vi "rs3 Get All Advanced3.vi"(7 "error in (no error)":errorcluster, 8 "device in":u64=370866768) -> (10 "ST_CensusEnable":cluster{"uDiameter":u32, "vDiameter":u32}={"uDiameter"=9, "vDiameter"=9}, 12 "ST_AE_Control":cluster{"meanIntensitySetpoint":u32}={"meanIntensitySetpoint"=400}, 14 "error":i32, 16 "Depth Table":T1={"depthUnits, um"=1000, "depthClampMin"=0, "depthClampMax"=65535, "disparityMultiplier"=0, "disparityShift"=0}, 17 "ST RAU vector":T7={"minWest"=1, "minEast"=1, "minWEsum"=1, "minNorth"=1, "minSouth"=1, "minNSSum"=1, "uStrink"=1, "vShrink"=1}, 18 "Dev out":u64=370866768, 19 "ST Color Control":T6, 20 "depth control":T2={"plusIncrement"=10, "MinusDecrement"=10, "deepSeaMedianThreshold"=528, "scoreThreshA"=10, "scoreThreshB"=1023, "textureDifferenceThreshold"=0, "textureCountThreshold"=0, "deepSeaSecondPeakThreshold"=27, "deepSeaNeighborThreshold"=20, "IrAgreeThreshold"=70}, 21 "STColorCorrection output":T9={"colorCorrection 1"=0.54785156, "colorCorrection 2"=0.32910156, "colorCorrection 3"=0.8222656, "colorCorrection 4"=0.109375, "colorCorrection 5"=-0.40527344, "colorCorrection 6"=-1.5253906, "colorCorrection 7"=0.95703125, "colorCorrection 8"=0.89160156, "colorCorrection 9"=0.7675781, "colorCorrection 10"=-0.4794922, "colorCorrection 11"=0.047851562, "colorCorrection 12"=-0.2705078}, 22 "HDAD":T10={"lambdaCensus"=26.0, "lambdaAD"=2100.0, "ignoreSAD"=0}, 23 "ST RSM":T8={"rsmBypass"=0, "diffThresh"=7.0, "sloRauDiffThresh"=3.0, "removeThresh"=33}, 24 "ST SLO Penalty":T3={"sloK1Penalty"=44, "sloK2Penalty"=502, "sloK1PenaltyMod1"=23, "sloK2PenaltyMod1"=237, "sloK1PenaltyMod2"=219, "sloK2PenaltyMod2"=113}, 25 "ST SLO Threshold":T4={"SLOdiffThresholdRed"=300, "SLODiffThresholdGreen"=300, "SLODiffThresholdBlue"=300}, 26 "ST Rau Threshold":T5={"rauDiffThresholdRed"=600, "rauDiffThresholdGreen"=600, "rauDiffThresholdBlue"=600}, 27 "error out":errorcluster)   [LabVIEW 2017, in "libRealSense3.lvlib"]
uses:
  libRealSense3.lvlib
panel:
  # "RS3 Get All Advanced"
  # "(C) 2017 Intel Corp.,  AGJ"
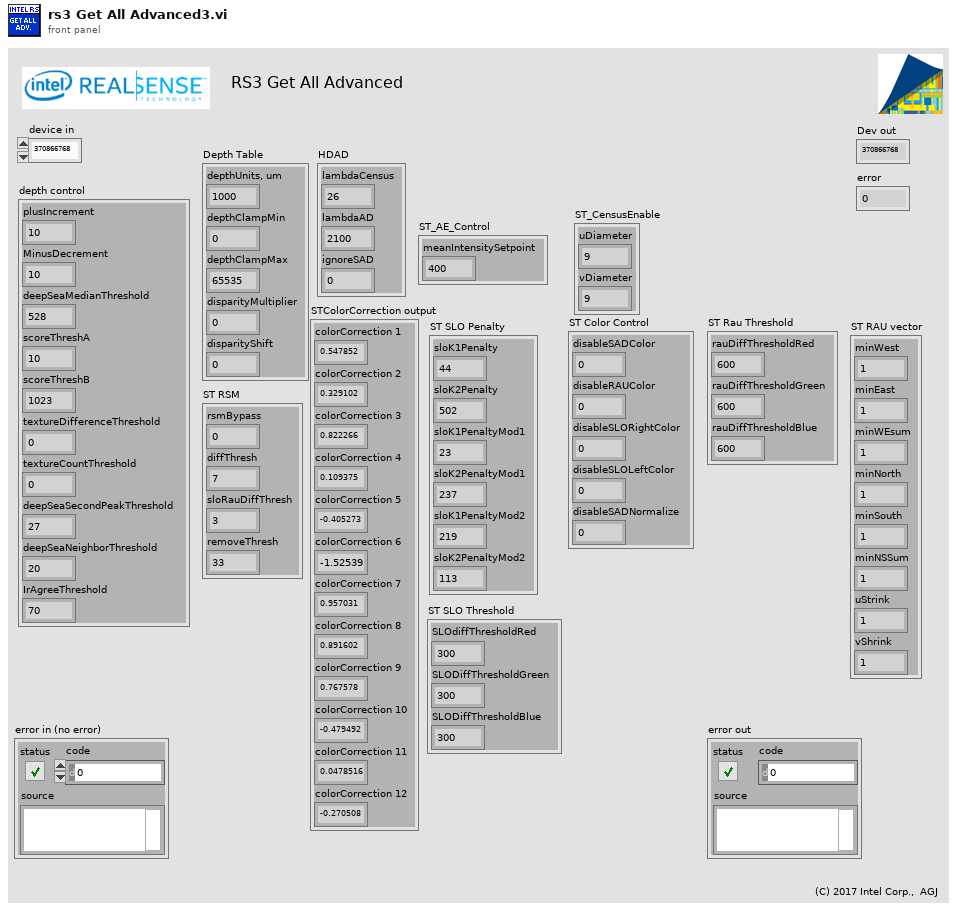
[diagram p1: front panel]
types:
  T1 = cluster{"depthUnits, um":u32, "depthClampMin":u32, "depthClampMax":u32, "disparityMultiplier":u32, "disparityShift":u32}
  T2 = cluster{"plusIncrement":u32, "MinusDecrement":u32, "deepSeaMedianThreshold":u32, "scoreThreshA":u32, "scoreThreshB":u32, "textureDifferenceThreshold":u32, "textureCountThreshold":u32, "deepSeaSecondPeakThreshold":u32, "deepSeaNeighborThreshold":u32, "IrAgreeThreshold":u32}
  T3 = cluster{"sloK1Penalty":u32, "sloK2Penalty":u32, "sloK1PenaltyMod1":u32, "sloK2PenaltyMod1":u32, "sloK1PenaltyMod2":u32, "sloK2PenaltyMod2":u32}
  T4 = cluster{"SLOdiffThresholdRed":u32, "SLODiffThresholdGreen":u32, "SLODiffThresholdBlue":u32}
  T5 = cluster{"rauDiffThresholdRed":u32, "rauDiffThresholdGreen":u32, "rauDiffThresholdBlue":u32}
  T6 = cluster{"disableSADColor":u32, "disableRAUColor":u32, "disableSLORightColor":u32, "disableSLOLeftColor":u32, "disableSADNormalize":u32}
  T7 = cluster{"minWest":u32, "minEast":u32, "minWEsum":u32, "minNorth":u32, "minSouth":u32, "minNSSum":u32, "uStrink":u32, "vShrink":u32}
  T8 = cluster{"rsmBypass":u32, "diffThresh":sgl, "sloRauDiffThresh":sgl, "removeThresh":u32}
  T9 = cluster{"colorCorrection 1":sgl, "colorCorrection 2":sgl, "colorCorrection 3":sgl, "colorCorrection 4":sgl, "colorCorrection 5":sgl, "colorCorrection 6":sgl, "colorCorrection 7":sgl, "colorCorrection 8":sgl, "colorCorrection 9":sgl, "colorCorrection 10":sgl, "colorCorrection 11":sgl, "colorCorrection 12":sgl}
  T10 = cluster{"lambdaCensus":sgl, "lambdaAD":sgl, "ignoreSAD":u32}
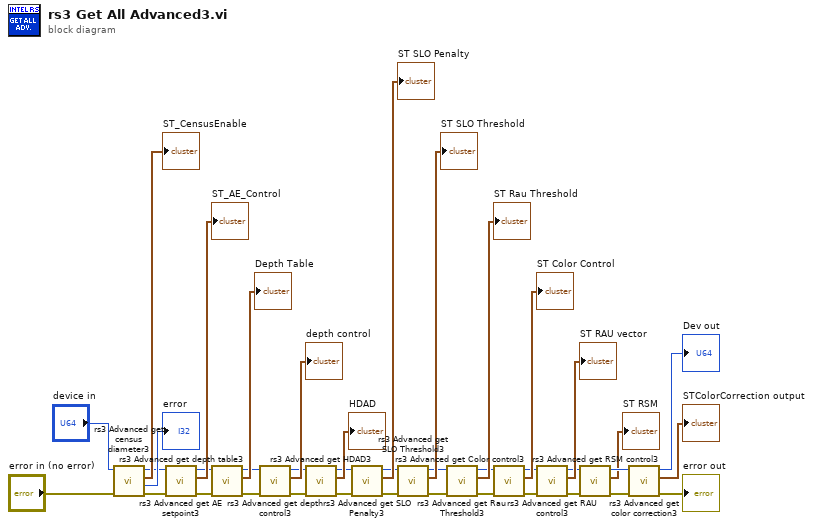
[diagram p0: block diagram]
diagram:
  n1 = call "rs3 Advanced get census diameter3.vi"("error in (no error)"="error in (no error)", "device in"="device in") -> ("error out 2"=w12:errorcluster, "error"=→"error":u64, "ST_CensusEnable"=→"ST_CensusEnable":cluster{"uDiameter":u32, "vDiameter":u32}, "Dev out"=w7:u64)  [unwired: 6 in]
  n2 = call "rs3 Advanced get AE setpoint3.vi"("error in (no error)"=w12, "device in"=w7) -> ("error out 2"=w8:errorcluster, "ST_AE_Control"=→"ST_AE_Control":cluster{"meanIntensitySetpoint":u32}, "Dev out"=w9:u64)  [unwired: 6 in, 1 out]
  n3 = call "rs3 Advanced get depth table3.vi"("error in (no error)"=w8, "device in"=w9) -> ("error out 2"=w3:errorcluster, "Depth Table"=→"Depth Table":T1, "Dev out"=w2:u64)  [unwired: 6 in, 1 out]
  n4 = call "rs3 Advanced get depth control3.vi"("error in (no error)"=w3, "device in"=w2) -> ("error out 2"=w38:errorcluster, "depth control"=→"depth control":T2, "Dev out"=w15:u64)  [unwired: 6 in, 1 out]
  n5 = call "rs3 Advanced get HDAD3.vi"("error in (no error)"=w38, "device in"=w15) -> ("error out 2"=w39:errorcluster, "HDAD"=→"HDAD":T10, "Dev out"=w16:u64)  [unwired: 6 in, 1 out]
  n6 = call "rs3 Advanced get SLO Penalty3.vi"("error in (no error)"=w39, "device in"=w16) -> ("error out 2"=w26:errorcluster, "ST SLO Penalty"=→"ST SLO Penalty":T3, "Dev out"=w17:u64)  [unwired: 6 in, 1 out]
  n7 = call "rs3 Advanced get SLO Threshold3.vi"("error in (no error)"=w26, "device in"=w17) -> ("error out 2"=w25:errorcluster, "ST SLO Threshold"=→"ST SLO Threshold":T4, "Dev out"=w18:u64)  [unwired: 6 in, 1 out]
  n8 = call "rs3 Advanced get Rau Threshold3.vi"("error in (no error)"=w25, "device in"=w18) -> ("error out 2"=w24:errorcluster, "ST Rau Threshold"=→"ST Rau Threshold":T5, "Dev out"=w19:u64)  [unwired: 6 in, 1 out]
  n9 = call "rs3 Advanced get Color control3.vi"("error in (no error)"=w24, "device in"=w19) -> ("error out 2"=w23:errorcluster, "ST Color Control"=→"ST Color Control":T6, "Dev out"=w20:u64)  [unwired: 6 in, 1 out]
  n10 = call "rs3 Advanced get RAU control3.vi"("error in (no error)"=w23, "device in"=w20) -> ("error out 2"=w22:errorcluster, "ST RAU vector"=→"ST RAU vector":T7, "Dev out"=w21:u64)  [unwired: 6 in, 1 out]
  n11 = call "rs3 Advanced get RSM control3.vi"("error in (no error)"=w22, "device in"=w21) -> ("error out 2"=w34:errorcluster, "ST RSM"=→"ST RSM":T8, "Dev out"=w35:u64)  [unwired: 6 in, 1 out]
  n12 = call "rs3 Advanced get color correction3.vi"("error in (no error)"=w34, "device in"=w35) -> ("error out 2"=→"error out":errorcluster, "STColorCorrection output"=→"STColorCorrection output":T9, "Dev out"=→"Dev out":u64)  [unwired: 6 in, 1 out]
